vi "addFile.vi"(8 "Error In":errorcluster, 10 "file":string, 11 "QIcon In":refnum<class "QIcon.lvclass">) -> (0 "Error Out":errorcluster, 3 "QIcon Out":refnum<class "QIcon.lvclass">)   [LabVIEW 2014, in "QIcon.lvclass"]
doc: "LabVIEW-specific documentation is not yet available. See <b>http://doc.qt.io/qt-5/QIcon.html#addFile</b>"
uses:
  QIcon.lvclass
  LQ Core/LQSerialData/LQSerialData.lvclass/LQSerialData.ctl
  LQ Core/LQ Core.lvlib
  LQ Core/LQSerialData/LQSerialData.lvclass
panel:
  # "Copyright (c) 2016 Sze Howe Koh\n\nThis Source Code Form is subject to the terms of the Mozilla Public\nLicense, v. 2.0. If a copy of the MPL was not distributed with this\nfile, You can obtain one at http://mozilla.org/MPL/2.0/."
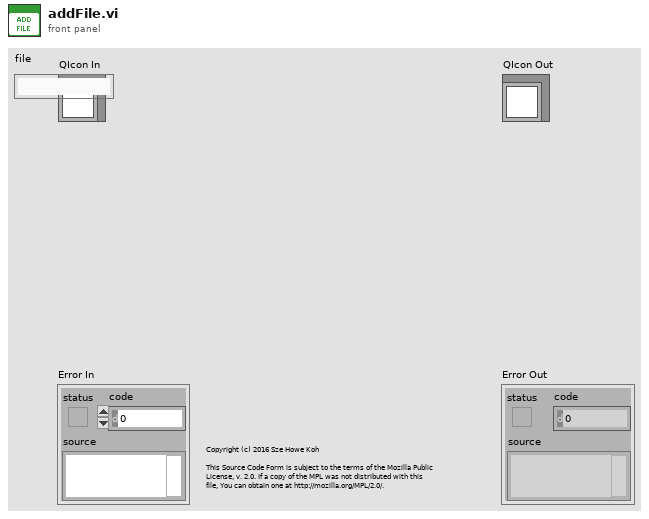
[diagram p1: front panel]
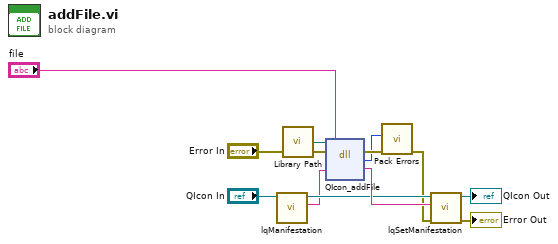
[diagram p0: block diagram]
diagram:
  n1 = call "lqManifestation.vi"("LQSerialData in"="QIcon In") -> ("Manifestation"=w7:string, "LQSerialData out"=w8:refnum<class "QIcon.lvclass">)  [unwired: 9 in]
  n2 = call "Library Path.vi"() -> ("Library Path"=w6:path)
  n3 = dll-call lib="?" fn="QIcon_addFile"(path in=w6, error in="Error In", "_instance"=w7, "file"="file") -> (error out=w5:errorcluster, w4:i32, "_instance"=w10:string)  [unwired: 2 in, 1 out]
  n4 = call "Pack Errors.vi"("Error In"=w5, "Error Code"=w4) -> ("Error Out"=w3:errorcluster)  [unwired: 9 in]
  n5 = call "lqSetManifestation.vi"("Error In"=w3, "Manifestation"=w10, "LQSerialData in"=w8) -> ("Error Out"=→"Error Out":errorcluster, "LQSerialData out"=→"QIcon Out":refnum<class "QIcon.lvclass">)  [unwired: 7 in]
